vi "Register gRPC Methods.vi"(8 "error in (no error)":errorcluster, 11 "Template Server in":refnum<class "dcvmDPI.lvclass">) -> (0 "error out":errorcluster, 3 "Template Server out":refnum<class "dcvmDPI.lvclass">)   [LabVIEW 2021, in "dcvmDPI_AD7606B_server.lvlib" / "dcvmDPI.lvclass"]
uses:
  dcvmDPI.lvclass
  typeDefs/Server Internal UEs.ctl
  typeDefs/Server Internal Message.ctl
  typeDefs/Server gRPC UEs.ctl
  <vilib>/gRPC/LabVIEW gRPC Library/Server API/typeDefs/gRPCId Cluster.ctl
  <vilib>/gRPC/LabVIEW gRPC Library/Shared/grpcId.ctl
  dcvmDPI.lvclass/dcvmDPI.ctl
  <vilib>/gRPC/LabVIEW gRPC Library/grpc-lvsupport-release.lvlib
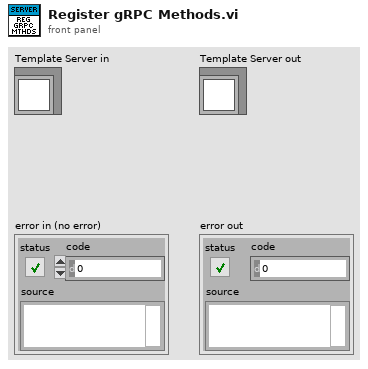
[diagram p1: front panel]
types:
  T1 = typedef "dcvmDPI_AD7606B_server.lvlib/dcvmDPI.lvclass/Server gRPC UEs.ctl" = cluster{"dcvmDPI ID gRPC UE":refnum<user-event>, "dcvmDPI ActiveMeasuresment gRPC UE":refnum<user-event>, "dcvmDPI Initialize gRPC UE":refnum<user-event>, "dcvmDPI Configure gRPC UE":refnum<user-event>, "dcvmDPI Initiate gRPC UE":refnum<user-event>, "dcvmDPI Acquire gRPC UE":refnum<user-event>, "dcvmDPI Close gRPC UE":refnum<user-event>}
  T2 = typedef "dcvmDPI_AD7606B_server.lvlib/dcvmDPI.lvclass/Server Internal UEs.ctl" = cluster{"dcvmDPI ID Internal UE":refnum<user-event>, "dcvmDPI ActiveMeasuresment Internal UE":refnum<user-event>, "dcvmDPI Initialize Internal UE":refnum<user-event>, "dcvmDPI Configure Internal UE":refnum<user-event>, "dcvmDPI Initiate Internal UE":refnum<user-event>, "dcvmDPI Acquire Internal UE":refnum<user-event>, "dcvmDPI Close Internal UE":refnum<user-event>}
  T3 = typedef "grpc-lvsupport-release.lvlib/grpcId.ctl" = u64
  T4 = typedef "dcvmDPI_AD7606B_server.lvlib/dcvmDPI.lvclass/Server Internal Message UE.ctl" = refnum<user-event>
  T5 = typedef "grpc-lvsupport-release.lvlib/gRPCId Cluster UE.ctl" = refnum<user-event>
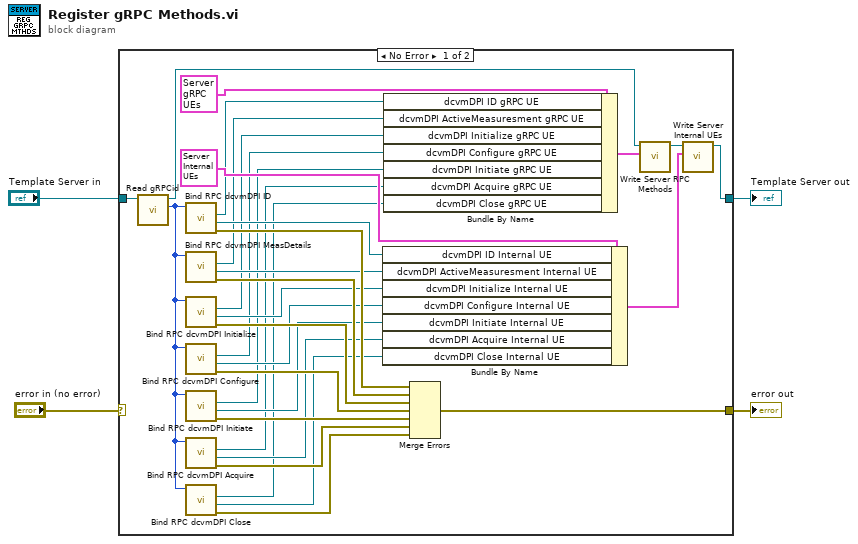
[diagram p0: block diagram]
diagram:
  n1 = case shown="No Error" "error in (no error)" {
    selector: "error in (no error)" -> [_ w36]
    tunnel: "Template Server in" -> [w27 w37]
    tunnel: [w35 w36] -> w3
    tunnel: [w34 w37] -> w2
    frame No Error {
      n2 = call-dynamic "Read gRPCid.vi"("iService in"=w27) -> ("gRPCid"=w26:T3, "iService out"=w28:refnum<class "dcvmDPI.lvclass">)  [unwired: 8 in, 1 out]
      n3 = call "Bind RPC dcvmDPI ID.vi"("gRPCid server in"=w26) -> ("error out"=w25:errorcluster, "dcvmDPI ID Internal UE"=w23:T4, "dcvmDPI ID gRPC UE"=w24:T5)  [unwired: 7 in, 1 out]
      n4 = call "Bind RPC dcvmDPI MeasDetails.vi"("gRPCid server in"=w26) -> ("error out"=w22:errorcluster, "dcvmDPI ActiveMeasuresment Internal UE"=w20:T4, "dcvmDPI ActiveMeasuresment gRPC UE"=w21:T5)  [unwired: 7 in, 1 out]
      n5 = call "Bind RPC dcvmDPI Initialize.vi"("gRPCid server in"=w26) -> ("error out"=w19:errorcluster, "dcvmDPI Initialize Internal UE"=w17:T4, "dcvmDPI Initialize gRPC UE"=w18:T5)  [unwired: 7 in, 1 out]
      n6 = call "Bind RPC dcvmDPI Configure.vi"("gRPCid server in"=w26) -> ("error out"=w16:errorcluster, "dcvmDPI Configure Internal UE"=w14:T4, "dcvmDPI Configure gRPC UE"=w15:T5)  [unwired: 7 in, 1 out]
      n7 = call "Bind RPC dcvmDPI Initiate.vi"("gRPCid server in"=w26) -> ("error out"=w13:errorcluster, "dcvmDPI Initiate Internal UE"=w11:T4, "dcvmDPI Initiate gRPC UE"=w12:T5)  [unwired: 7 in, 1 out]
      n8 = call "Bind RPC dcvmDPI Acquire.vi"("gRPCid server in"=w26) -> ("error out"=w10:errorcluster, "dcvmDPI Acquire Internal UE"=w8:T4, "dcvmDPI Acquire gRPC UE"=w9:T5)  [unwired: 7 in, 1 out]
      n9 = call "Bind RPC dcvmDPI Close.vi"("gRPCid server in"=w26) -> ("error out"=w7:errorcluster, "dcvmDPI Close Internal UE"=w5:T4, "dcvmDPI Close gRPC UE"=w6:T5)  [unwired: 7 in, 1 out]
      n10 = Bundle By Name ("Bundle Internal UEs")(cluster=T2 {"dcvmDPI ID Internal UE"=refnum, "dcvmDPI ActiveMeasuresment Internal UE"=refnum, "dcvmDPI Initialize Internal UE"=refnum, "dcvmDPI Configure Internal UE"=refnum, "dcvmDPI Initiate Internal UE"=refnum, "dcvmDPI Acquire Internal UE"=refnum, "dcvmDPI Close Internal UE"=refnum} ("Server Internal UEs"), "dcvmDPI ID Internal UE"=w23, "dcvmDPI ActiveMeasuresment Internal UE"=w20, "dcvmDPI Initialize Internal UE"=w17, "dcvmDPI Configure Internal UE"=w14, "dcvmDPI Initiate Internal UE"=w11, "dcvmDPI Acquire Internal UE"=w8, "dcvmDPI Close Internal UE"=w5) -> (w33:T2)
      n11 = Bundle By Name ("Bundle gRPC UEs")(cluster=T1 {"dcvmDPI ID gRPC UE"=refnum, "dcvmDPI ActiveMeasuresment gRPC UE"=refnum, "dcvmDPI Initialize gRPC UE"=refnum, "dcvmDPI Configure gRPC UE"=refnum, "dcvmDPI Initiate gRPC UE"=refnum, "dcvmDPI Acquire gRPC UE"=refnum, "dcvmDPI Close gRPC UE"=refnum} ("gRPC Server Method Events"), "dcvmDPI ID gRPC UE"=w24, "dcvmDPI ActiveMeasuresment gRPC UE"=w21, "dcvmDPI Initialize gRPC UE"=w18, "dcvmDPI Configure gRPC UE"=w15, "dcvmDPI Initiate gRPC UE"=w12, "dcvmDPI Acquire gRPC UE"=w9, "dcvmDPI Close gRPC UE"=w6) -> (w30:T1)
      n12 = Merge Errors(w25, w22, w19, w16, w13, w10, w7) -> (w35:errorcluster)
      n13 = call "Write Server RPC Methods.vi"("Server RPC Methods"=w30, "SignalGeneratorService in"=w28) -> ("SignalGeneratorService out"=w31:refnum<class "dcvmDPI.lvclass">)  [unwired: 8 in, 1 out]
      n14 = call "Write Server Internal UEs.vi"("Server Internal UEs"=w33, "SignalGeneratorService in"=w31) -> ("SignalGeneratorService out"=w34:refnum<class "dcvmDPI.lvclass">)  [unwired: 8 in, 1 out]
    }
    frame Error {
    }
  }
  "error out" <- w3
  "Template Server out" <- w2
